vi "MainFlow_Monitor.vi"(11 "VISA resource name":refnum<visa-resource-name>) -> (0 "Error at segmenting output":errorcluster, 1 "Error at VISA Read":errorcluster, 3 "Flow readout":dbl)   [LabVIEW 2015]
uses:
  <vilib>/Utility/config.llb/Read Key (I32).vi
  <vilib>/Utility/file.llb/Write Delimited Spreadsheet (DBL).vi
  <vilib>/Utility/config.llb/NI_LVConfig.lvlib
panel:
  out "Waveform Chart 2":dbl(graph)
  out "date/time string 2":string
  out "current time 2":timestamp
  out "decimal integer string":string
  out "remaining string":string
  out "read buffer":string
  out "result":bool
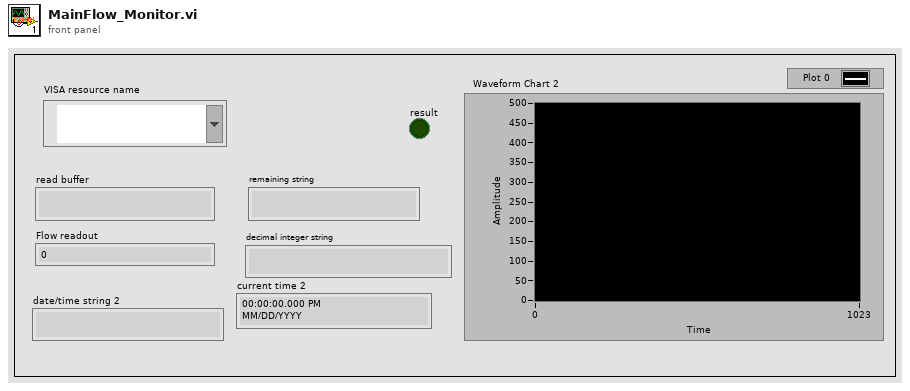
[diagram p1: front panel]
types:
  T1 = typedef "NI_LVConfig.lvlib/Config Data RefNum.ctl" = refnum<k1>
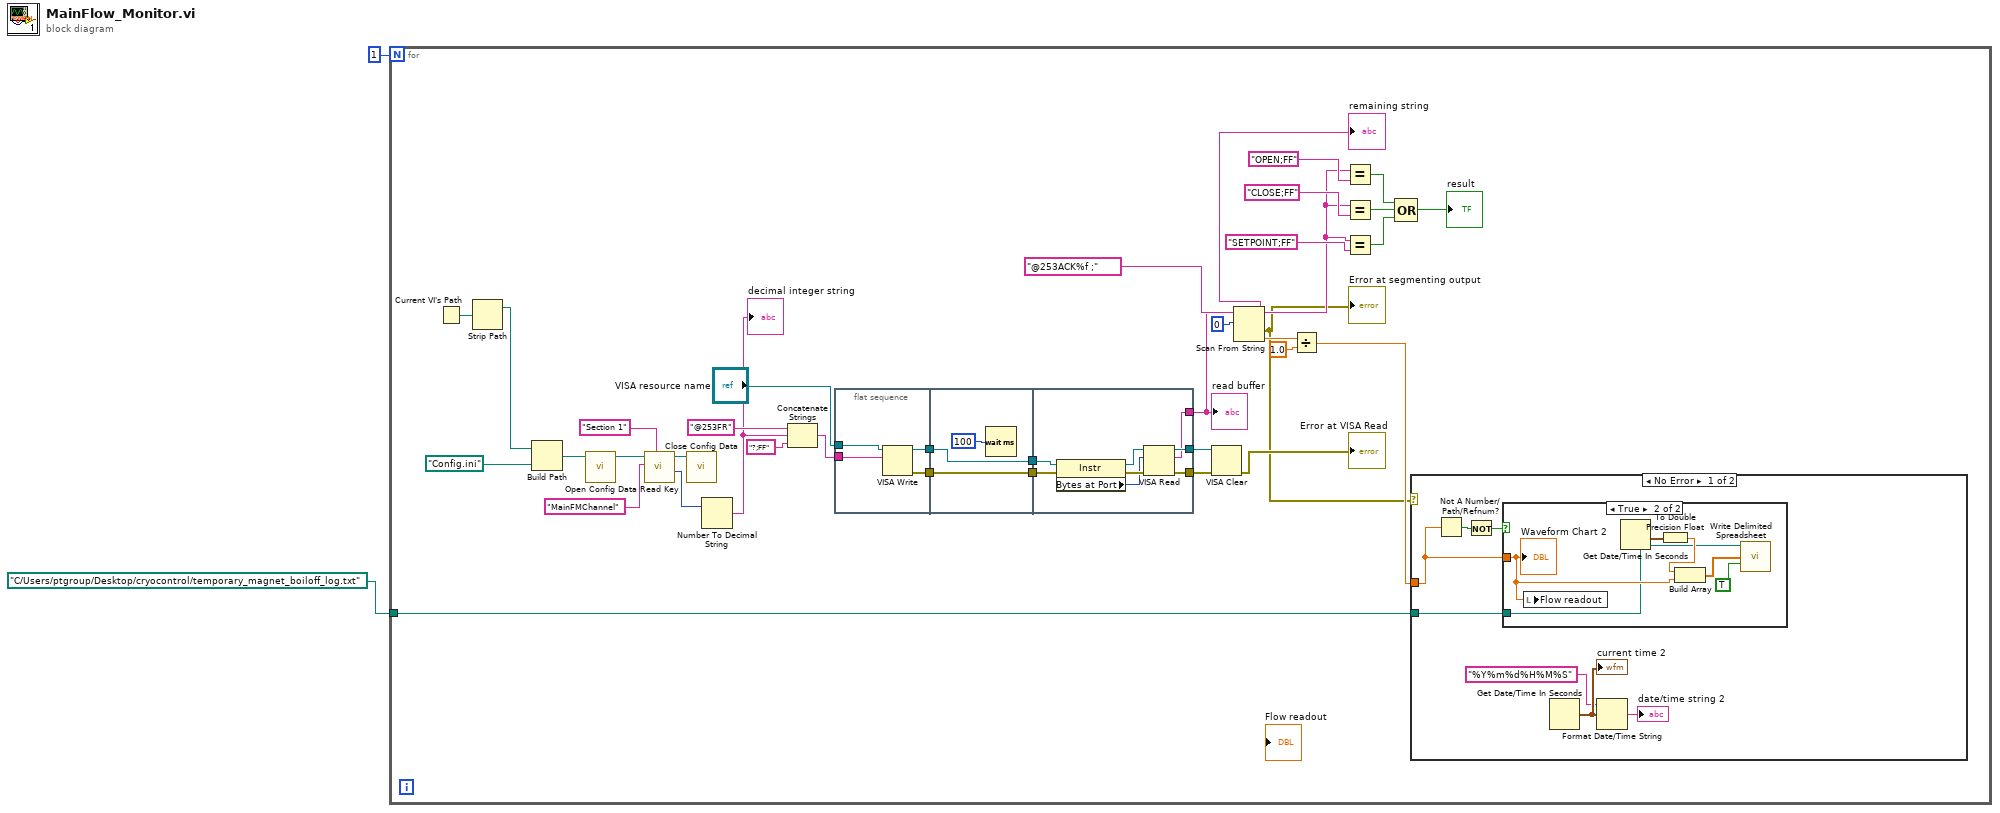
[diagram p0: block diagram]
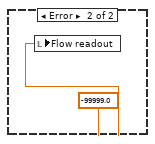
[diagram p3: hidden frame]
diagram:
  n1 = for {
    N: 1 -> [_]
    tunnel: path "C:/Users/ptgroup/Desktop/cryocontrol/temporary_magnet_boiloff_log.txt" ("default name") -> [w3]
    n2 = Current VI's Path() -> (path=w5:path)
    n3 = Strip Path(path=w5) -> (stripped path=w4:path)  [unwired: 1 out]
    n4 = Build Path(base path=w4, name or relative path=path "Config.ini" ("default name")) -> (appended path=w28:path)
    n5 = call <vilib>:"Open Config Data.vi"("configuration file path"=w28) -> ("refnum"=w35:T1)  [unwired: 8 in, 2 out]
    n6 = call-poly <vilib>:"Read Key.vi"("section"="Section 1", "key"="MainFMChannel", "refnum"=w35) -> ("value"=w32:i32, "refnum out"=w33:T1)  [unwired: 5 in, 2 out]
    n7 = call <vilib>:"Close Config Data.vi"("refnum"=w33) -> ()  [unwired: 9 in, 2 out]
    n8 = Number To Decimal String(number=w32) -> (decimal integer string=w30:string)  [unwired: 1 in]
    "decimal integer string" <- w30
    n9 = Concatenate Strings("@253FR" ("string"), w30, "?;FF" ("string")) -> (w14:string)
    n10 = flat-sequence {
      tunnel: w14 -> [w43]
      tunnel: "VISA resource name" -> [w42]
      tunnel: [w41] -> w12
      tunnel: [w40] -> w10
      tunnel: w12 -> [w45]
      tunnel: [w45] -> w11
      tunnel: w10 -> [w44]
      tunnel: [w44] -> w9
      tunnel: w11 -> [w51]
      tunnel: w9 -> [w50]
      tunnel: [w49] -> w8
      tunnel: [w48] -> w6
      tunnel: [w47] -> w7
      frame #0 {
        n11 = VISA Write(VISA resource name=w42, write buffer=w43) -> (VISA resource name out=w41:refnum<visa-resource-name>, error out=w40:errorcluster)  [unwired: 1 in, 1 out]
      }
      frame #1 {
        n12 = Wait (ms)(milliseconds to wait=u32 100) -> ()  [unwired: 1 out]
      }
      frame #2 {
        n13 = property class="Instr"(reference=w51, error in=w50) -> (reference out=w52:refnum<visa-resource-name>, error out=w54:errorcluster, "Bytes at Port"=w53:u32)
        n14 = VISA Read(VISA resource name=w52, byte count=w53, error in (no error)=w54) -> (VISA resource name out=w49:refnum<visa-resource-name>, read buffer=w47:string, error out=w48:errorcluster)  [unwired: 1 out]
      }
    }
    n15 = VISA Clear(VISA resource name=w8, error in (no error)=w6) -> (error out=→"Error at VISA Read":errorcluster)  [unwired: 1 out]
    n16 = Scan From String(format string="@253ACK%f ;", input string=w7, initial scan location=u32 0) -> (remaining string=w18:string, error out=w15:errorcluster, output 1=w26:dbl)  [unwired: 2 in, 1 out]
    "Error at segmenting output" <- w15
    "remaining string" <- w18
    n17 = Divide(x=w26, y=1.0) -> (x/y=w25:dbl)
    n18 = Equal?(x=w18, y="OPEN;FF") -> (x = y?=w23:bool)
    n19 = Equal?(x=w18, y="CLOSE;FF") -> (x = y?=w22:bool)
    n20 = Equal?(x=w18, y="SETPOINT;FF") -> (x = y?=w19:bool)
    n21 = Compound Arithmetic op=OR(w23, w22, w19) -> (→"result":bool)
    n22 = case shown="No Error" w15 {
      tunnel: w25 -> [w57 _]
      tunnel: w3 -> [w55 _]
      frame No Error {
        n23 = Not A Number/Path/Refnum?(number/path/refnum=w57) -> (NaN/Path/Refnum?=w59:bool)
        n24 = Not(x=w59) -> (.not. x?=w58:bool)
        n25 = case shown="True" w58 {
          tunnel: w57 -> [_ w65]
          tunnel: w55 -> [_ w63]
          frame False {
          }
          frame True {
            n26 = local write "Flow readout"(w65) -> ()
            n27 = Get Date/Time In Seconds() -> (seconds since 1Jan1904=w66:timestamp)
            n28 = To Double Precision Float(number=w66) -> (double precision float=w67:dbl)
            n29 = Build Array(w67, w65) -> (w62:dbl[])
            n30 = call-poly <vilib>:"Write Delimited Spreadsheet.vi"("file path (dialog if empty)"=w63, "1D data"=w62, "append to file? (F)"=TRUE) -> ()  [unwired: 11 in, 2 out]
            "Waveform Chart 2" <- w65
          }
        }
        n31 = Get Date/Time In Seconds() -> (seconds since 1Jan1904=w61:timestamp)
        "current time 2" <- w61
        n32 = Format Date/Time String(time format string (%c)="%Y%m%d%H%M%S", seconds (now)=w61) -> (date/time string=→"date/time string 2":string)  [unwired: 1 in]
      }
      frame Error {
        n33 = local write "Flow readout"(-99999.0) -> ()
      }
    }
    "read buffer" <- w7
  }
